vi "Get Status.vi"(8 "error in (no error)":errorcluster, 11 "DM-SetPower-Command in":refnum<class "DM-SetPower-Command.lvclass">) -> (0 "error out":errorcluster, 2 "Status":string, 3 "DM-SetPower-Command out":refnum<class "DM-SetPower-Command.lvclass">)   [LabVIEW 2013, in "DM-SetPower-Command.lvclass"]
uses:
  DM-SetPower-Command.lvclass
  Command/Command.lvclass
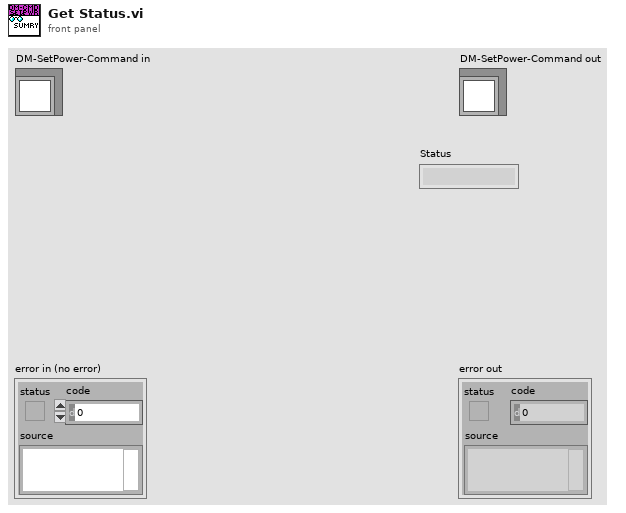
[diagram p1: front panel]
types:
  T1 = typedef "DM-SetPower-Command.lvclass/DM-SetPower-Command-Arguments.ctl" = cluster{"Power":dbl}
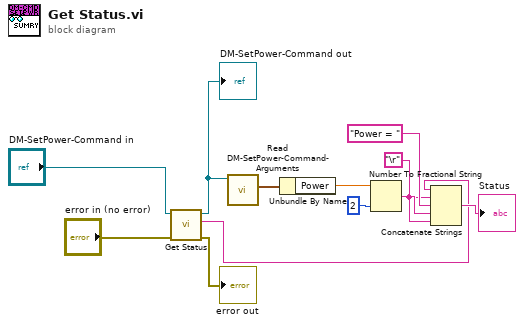
[diagram p0: block diagram]
diagram:
  w3 = "\r"
  n1 = call-parent "Get Status.vi"("error in (no error)"="error in (no error)", "Command in"="DM-SetPower-Command in") -> ("error out"=→"error out":errorcluster, "Status"=w1:string, "Command out"=w4:refnum<class "DM-SetPower-Command.lvclass">)  [unwired: 7 in]
  "DM-SetPower-Command out" <- w4
  n2 = call-dynamic "Read DM-SetPower-Command-Arguments.vi"("DM-SetPower-Command in"=w4) -> ("DM-SetPower-Command-In"=w7:T1)  [unwired: 8 in, 2 out]
  n3 = Unbundle By Name(w7) -> ("Power"=w6:dbl)
  n4 = Number To Fractional String(number=w6, precision (6)=i16 2 ("width (-)")) -> (F-format string=w5:string)  [unwired: 2 in]
  n5 = Concatenate Strings(w1, w3, "Power = ", w5, w3) -> (→"Status":string)
